vi "Paramatrized.vi"(11 "column information":T1[](array[typedef])=[{"column name"="Signal_x", "data type"=enum."Double (DBL)", "size"=0, "allow null?"=TRUE}, {"column name"="Signal_y", "data type"=enum."Double (DBL)", "size"=0, "allow null?"=TRUE}, {"column name"="Signal_z", "data type"=enum."Double (DBL)", "size"=0, "allow null?"=TRUE}]) -> (3 "parameters":T3[](array[typedef]))   [LabVIEW 2019]
uses:
  <vilib>/addons/database/Auxilliary.llb/DB Tools Parameter Info.ctl
  <vilib>/addons/database/Auxilliary.llb/DB Tools DataTypes.ctl
  <vilib>/addons/database/Auxilliary.llb/DB Tools Parameter Dir.ctl
  <vilib>/addons/database/Auxilliary.llb/DB Tools Column Info.ctl
  <vilib>/addons/database/NI_Database_API.lvlib
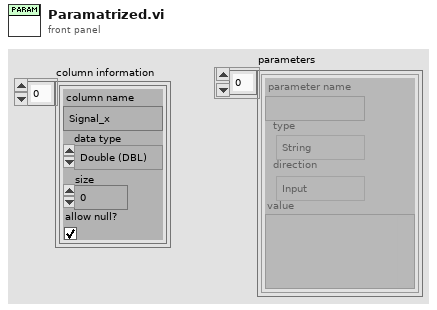
[diagram p1: front panel]
types:
  T1 = typedef "NI_Database_API.lvlib/DB Tools Column Info.ctl" = cluster{"column name":string, "data type":T2, "size":i32, "allow null?":bool}
  T2 = typedef "NI_Database_API.lvlib/DB Tools DataTypes.ctl" = enum16{"String", "Long (I32)", "Single (SGL)", "Double (DBL)", "Date/Time", "Binary"}
  T3 = typedef "NI_Database_API.lvlib/DB Tools Parameter Info.ctl" = cluster{"parameter name":string, "type":T2, "direction":T4, "value":variant}
  T4 = typedef "NI_Database_API.lvlib/DB Tools Parameter Dir.ctl" = enum32{"Input", "Output", "Input/Output", "Return Value"}
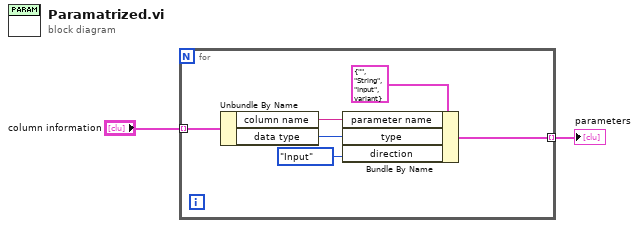
[diagram p0: block diagram]
diagram:
  n1 = for {
    tunnel: "column information" -> [w7] mode=indexing
    tunnel: [w3] -> w2 mode=indexing
    n2 = Unbundle By Name(w7) -> ("column name"=w6:string, "data type"=w5:T2)
    n3 = Bundle By Name(cluster=T3 {"parameter name"="", "type"=enum."String", "direction"=enum."Input", "value"=variant} ("parameter information"), "parameter name"=w6, "type"=w5, "direction"=DB_Tools_Parameter_Dir."Input") -> (w3:T3)
  }
  "parameters" <- w2
